vi "read_once.vi"() -> ()   [LabVIEW 2014]
uses:
  <instrlib>/Hokuyo URG Series/Public/Initialize-Standard.vi
  <vilib>/Instr/_visa.llb/VISA Configure Serial Port (Instr).vi
  <vilib>/Utility/file.llb/Write To Spreadsheet File (DBL).vi
  <instrlib>/Hokuyo URG Series/Hokuyo URG Series.lvlib
panel:
  in  "Stop":dbl
  in  "Step":dbl
  in  "VISA resource name":refnum<visa-resource-name>
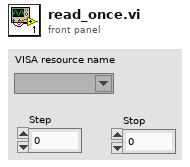
[diagram p1: front panel]
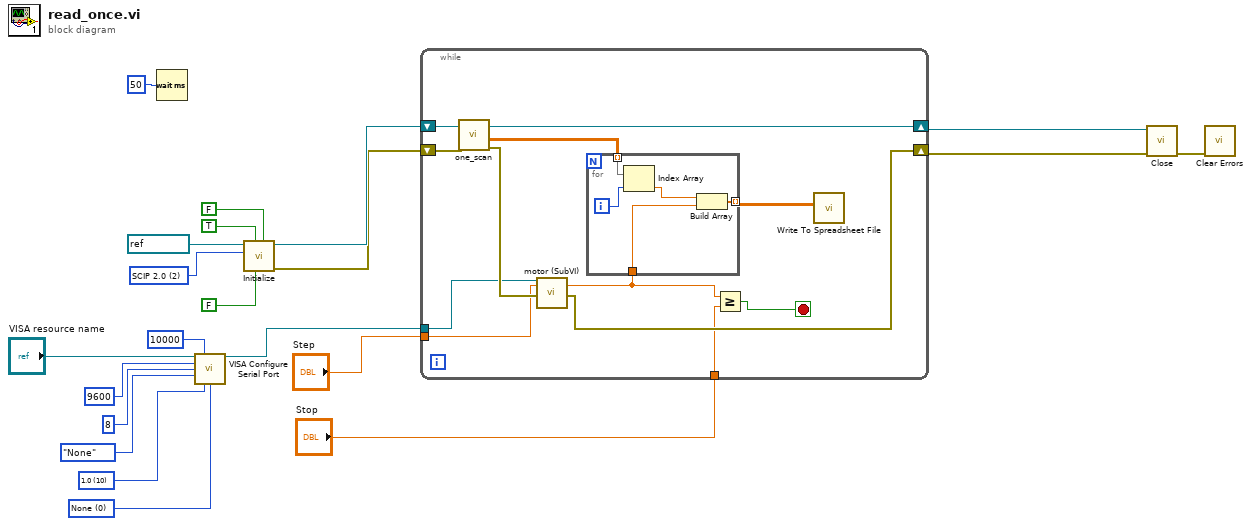
[diagram p0: block diagram]
diagram:
  w3 = u16 0 items=["None", "XON/XOFF", "RTS/CTS", "XON/XOFF & RTS/CTS", "DTR/DSR", "XON/XOFF & DTR/DSR"] ("flow control (0:none)")
  w4 = u16 10 items=["1.0"=10, "1.5"=15, "2.0"=20] ("stop bits (10: 1 bit)")
  w17 = u32 2 items=["Convert to Latest", "SCIP 1.1", "SCIP 2.0"] ("Protocol")
  n1 = Wait (ms)(milliseconds to wait=u32 50) -> ()  [unwired: 1 out]
  n2 = call-poly "VISA Configure Serial Port"("VISA resource name"="VISA resource name", "timeout (10sec)"=u32 10000, "baud rate (9600)"=u32 9600, "data bits (8)"=u16 8, "parity (0:none)"=enum16{"None", "Odd", "Even", "Mark", "Space"}."None", "stop bits (10: 1 bit)"=w4, "flow control (0:none)"=w3) -> ("VISA resource name out"=w10:refnum<visa-resource-name>)  [unwired: 7 in, 1 out]
  n3 = call-poly <instrlib>:"Initialize.vi"("Reset? (F: No)"=FALSE ("Reset Instrument (Disabled)"), "Checksum (Disabled)"=FALSE ("Checksum"), "ID Query? (Enabled)"=TRUE ("ID Query?"), "Protocol (2: SCIP 2.0)"=w17, "VISA resource name"=refnum<visa-resource-name> "COM3") -> ("error out"=w14:errorcluster, "VISA resource name out"=w15:refnum<visa-resource-name>)  [unwired: 5 in]
  n4 = while {
    tunnel: w10 -> [w28]
    tunnel: "Step" -> [w29]
    shift-right: [w33] -> w16
    shift-left: w15 -> [w32]
    shift-right: [w27] -> w21
    shift-left: w14 -> [w31]
    tunnel: "Stop" -> [w23]
    stop <- w24 stop-if-true
    n5 = call "one_scan.vi"("error in (no error)"=w31, "VISA Refnum in"=w32) -> ("error out"=w30:errorcluster, "PhiR Array"=w26:dbl[][], "VISA Refnum out"=w33:refnum<visa-resource-name>)  [unwired: 6 in, 1 out]
    n6 = call "motor (SubVI).vi"("VISA Refnum in"=w28, "step"=w29, "error in (no error)"=w30) -> ("Angle"=w22:dbl, "error out"=w27:errorcluster)  [unwired: 14 in, 1 out]
    n7 = for {
      tunnel: w26 -> [w38] mode=indexing
      tunnel: [w35] -> w25 mode=indexing
      tunnel: w22 -> [w34]
      i -> [w37]
      n8 = Index Array(array=w38, index=w37) -> (element=w36:dbl)
      n9 = Build Array(w36, w34) -> (w35:dbl[])
    }
    n10 = Greater Or Equal?(x=w22, y=w23) -> (x >= y?=w24:bool)
    n11 = call-poly <vilib>:"Write To Spreadsheet File.vi"("2D data"=w25) -> ()  [unwired: 7 in, 1 out]
  }
  n12 = call <instrlib>:"Close.vi"("error in (no error)"=w21, "VISA resource name"=w16) -> ("error out"=w12:errorcluster)  [unwired: 9 in]
  n13 = call <vilib>:"Clear Errors.vi"("error in (no error)"=w12) -> ()  [unwired: 5 in, 2 out]
